vi "BIO_set_tcp_ndelay.vi"(8 "error in (no error)":errorcluster, 10 "No Delay?":bool=TRUE, 11 "BIO in":refnum<class "BIO.lvclass">) -> (0 "error out":errorcluster, 3 "BIO out":refnum<class "BIO.lvclass">)   [LabVIEW 2013, in "OpenSSL Socket.lvlib" / "BIO.lvclass"]
uses:
  BIO.lvclass
  SSL-Lib/SSL-Lib.lvclass/SSL-Lib.ctl
  SSL-Lib/Read Crypto Library Path.vi
  SSL-Lib/SSL-Lib.lvclass
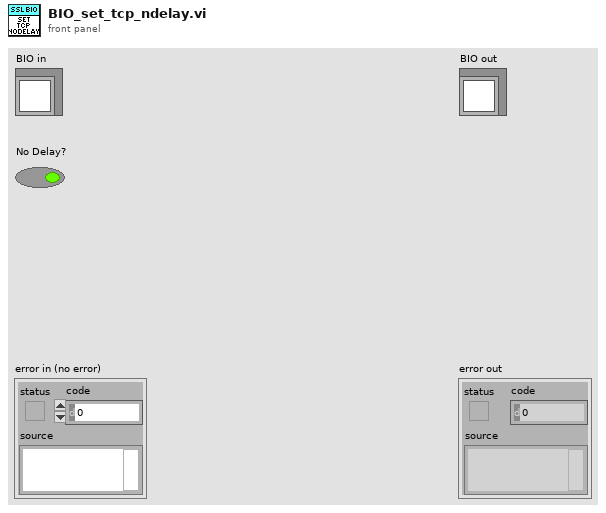
[diagram p1: front panel]
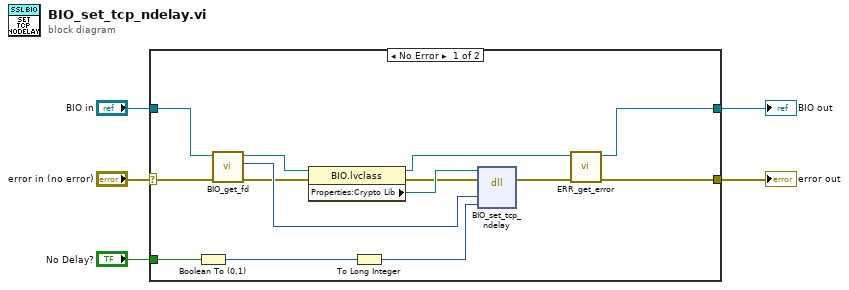
[diagram p0: block diagram]
diagram:
  n1 = case shown="No Error" "error in (no error)" {
    selector: "error in (no error)" -> [w11 w21]
    tunnel: [w17 w21] -> w4
    tunnel: [w16 w20] -> w2
    tunnel: "BIO in" -> [w10 w20]
    tunnel: "No Delay?" -> [w15 _]
    frame No Error {
      n2 = Boolean To (0,1)(Boolean=w15) -> (0, 1=w14:i16)
      n3 = call "BIO_get_fd.vi"("error in (no error)"=w11, "BIO in"=w10) -> ("error out"=w8:errorcluster, "socket fd"=w12:i32, "BIO out"=w9:refnum<class "BIO.lvclass">)  [unwired: 7 in]
      n4 = property class="BIO.lvclass"(reference=w9, error in=w8) -> (reference out=w6:refnum<class "BIO.lvclass">, error out=w7:errorcluster, "Properties:Crypto Lib"=w19:path)
      n5 = To Long Integer(number=w14) -> (32bit integer=w13:i32)
      n6 = dll-call lib="C:/Program Files (x86)/National Instruments/Shared/nissl/NIlibeay32.dll" fn="BIO_set_tcp_ndelay"(path in=w19, error in=w7, "sock"=w12, "turn_on"=w13) -> (error out=w18:errorcluster)  [unwired: 4 in, 1 out]
      n7 = call "ERR_get_error.vi"("error in (no error)"=w18, "SSL-Lib in"=w6) -> ("error out"=w17:errorcluster, "SSL-Lib out"=w16:refnum<class "BIO.lvclass">)  [unwired: 8 in]
    }
    frame Error {
    }
  }
  "error out" <- w4
  "BIO out" <- w2
